vi "Run All.vi"(8 "Error In":errorcluster) -> (0 "Error Out":errorcluster)   [LabVIEW 2017, in "Tests.lvlib" / "Version.lvlib"]
uses:
  Version.lvlib
  <vilib>/addons/_JKI Toolkits/Caraya/classes/Test/Test.lvclass
  src/LabPack/LabPack.lvlib
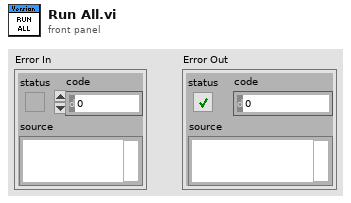
[diagram p1: front panel]
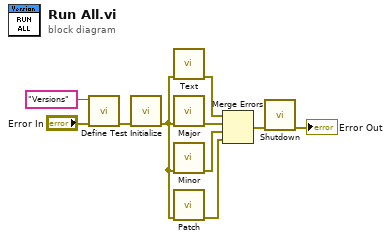
[diagram p0: block diagram]
diagram:
  n1 = call <vilib>:"Define Test.vi"("error in (no error)"="Error In", "Label (VI Title)"="Versions") -> ("error out"=w4:errorcluster)  [unwired: 9 in]
  n2 = call "Initialize.vi"("Error In"=w4) -> ("Error Out"=w3:errorcluster)  [unwired: 9 in, 1 out]
  n3 = call "Text.vi"("Error In"=w3) -> ("Error Out"=w10:errorcluster)  [unwired: 10 in]
  n4 = call "Major.vi"("Error In"=w3) -> ("Error Out"=w9:errorcluster)  [unwired: 10 in]
  n5 = call "Minor.vi"("Error In"=w3) -> ("Error Out"=w8:errorcluster)  [unwired: 10 in]
  n6 = call "Patch.vi"("Error In"=w3) -> ("Error Out"=w7:errorcluster)  [unwired: 10 in]
  n7 = Merge Errors(w10, w9, w8, w7) -> (w2:errorcluster)
  n8 = call "Shutdown.vi"("Error In"=w2) -> ("Error Out"=→"Error Out":errorcluster)  [unwired: 10 in]
